vi "write-attributes.vi"(7 "name":string="pressure", 8 "error in (no error)":errorcluster, 11 "ref in":T1 format="%.0x") -> (0 "error out":errorcluster, 3 "ref out":T1 format="%.0x")   [LabVIEW 2016]
uses:
  <vilib>/addons/h5labview2/base/hid_t.ctl
  <vilib>/addons/h5labview2/base/lib_path.vi
  <vilib>/addons/h5labview2/base/H5Equery.vi
  <vilib>/addons/h5labview2/attrib/H5Awrite.llb/H5Awrite.xnode
  <vilib>/addons/h5labview2/attrib/H5A.lvlib
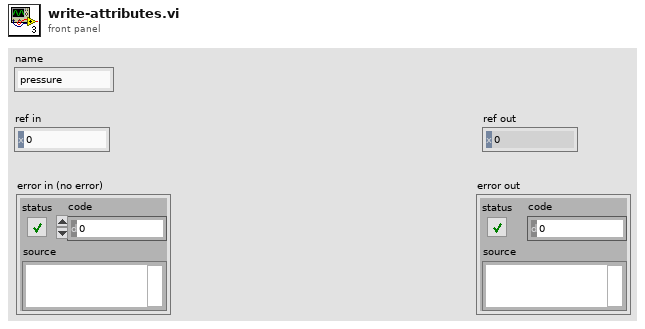
[diagram p1: front panel]
types:
  T1 = typedef "hid_t.ctl" = i32
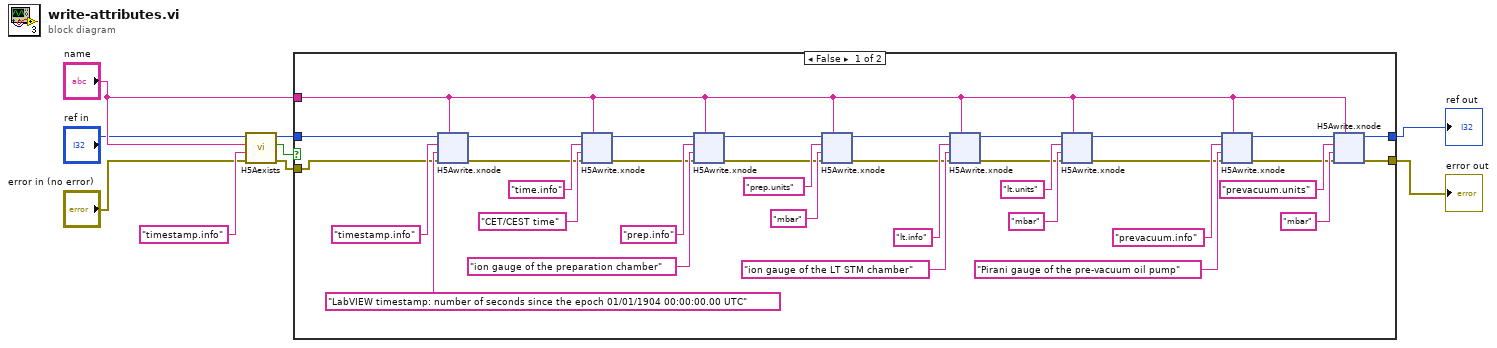
[diagram p0: block diagram]
diagram:
  n1 = call <vilib>:"H5Aexists.vi"("error in (no error)"="error in (no error)", "name"="timestamp.info" ("attrib name"), "object (.)"="name", "ref in"="ref in") -> ("error out"=w8:errorcluster, "exists?"=w5:bool, "ref out"=w7:T1)  [unwired: 5 in]
  n2 = case shown="False" w5 {
    tunnel: w7 -> [w28 w198]
    tunnel: w8 -> [w27 w197]
    tunnel: [w18 w198] -> w2
    tunnel: [w17 w197] -> w9
    tunnel: "name" -> [w10 _]
    frame False {
      n3 = xnode "H5Awrite.xnode"("object name"=w10, "error in (no error)"=w27, "data"="LabVIEW timestamp: number of seconds since the epoch 01/01/1904 00:00:00.00 UTC" ("attrib name"), "attrib name"="timestamp.info", "ref in"=w28) -> ("error out"=w11:errorcluster, "ref out"=w14:i32)  [unwired: 2 in, 1 out]
      n4 = xnode "H5Awrite.xnode"("object name"=w10, "error in (no error)"=w11, "data"="CET/CEST time" ("attrib name"), "attrib name"="time.info", "ref in"=w14) -> ("error out"=w12:errorcluster, "ref out"=w13:i32)  [unwired: 2 in, 1 out]
      n5 = xnode "H5Awrite.xnode"("object name"=w10, "error in (no error)"=w12, "data"="ion gauge of the preparation chamber" ("attrib name"), "attrib name"="prep.info", "ref in"=w13) -> ("error out"=w39:errorcluster, "ref out"=w40:i32)  [unwired: 2 in, 1 out]
      n6 = xnode "H5Awrite.xnode"("object name"=w10, "error in (no error)"=w39, "data"="mbar" ("attrib name"), "attrib name"="prep.units", "ref in"=w40) -> ("error out"=w24:errorcluster, "ref out"=w26:i32)  [unwired: 2 in, 1 out]
      n7 = xnode "H5Awrite.xnode"("object name"=w10, "error in (no error)"=w24, "data"="ion gauge of the LT STM chamber" ("attrib name"), "attrib name"="lt.info", "ref in"=w26) -> ("error out"=w23:errorcluster, "ref out"=w25:i32)  [unwired: 2 in, 1 out]
      n8 = xnode "H5Awrite.xnode"("object name"=w10, "error in (no error)"=w23, "data"="mbar" ("attrib name"), "attrib name"="lt.units", "ref in"=w25) -> ("error out"=w21:errorcluster, "ref out"=w22:i32)  [unwired: 2 in, 1 out]
      n9 = xnode "H5Awrite.xnode"("object name"=w10, "error in (no error)"=w21, "data"="Pirani gauge of the pre-vacuum oil pump" ("attrib name"), "attrib name"="prevacuum.info", "ref in"=w22) -> ("error out"=w19:errorcluster, "ref out"=w20:i32)  [unwired: 2 in, 1 out]
      n10 = xnode "H5Awrite.xnode"("object name"=w10, "error in (no error)"=w19, "data"="mbar" ("attrib name"), "attrib name"="prevacuum.units", "ref in"=w20) -> ("error out"=w17:errorcluster, "ref out"=w18:i32)  [unwired: 2 in, 1 out]
    }
    frame True {
    }
  }
  "error out" <- w9
  "ref out" <- w2
